vi "IO Manager.vi"(5 "Reentrant?":bool, 7 "Actions":T4, 11 "Mutex Name":string) -> (3 "Success?":bool)   [LabVIEW 2021]
uses:
  <vilib>/myRIO/Common/Instrument Driver Framework/Utilities/typedefs/Resource Manager Action Enum.ctl
  <vilib>/myRIO/Common/Instrument Driver Framework/Utilities/typedefs/Mutex Collection.ctl
  <vilib>/myRIO/Common/Instrument Driver Framework/Utilities/typedefs/Named Mutex.ctl
  <vilib>/myRIO/Common/Instrument Driver Framework/Utilities/typedefs/Reentrant Mutex.ctl
panel:
  out "Mutex Collection":T1
  out "error out":errorcluster
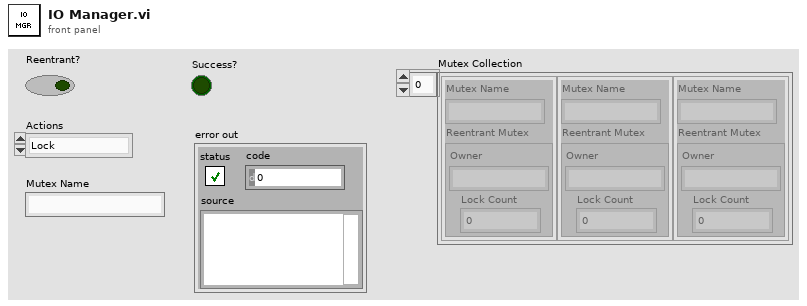
[diagram p1: front panel]
types:
  T1 = typedef "Mutex Collection.ctl" = T2[]
  T2 = typedef "Named Mutex.ctl" = cluster{"Mutex Name":string, "Reentrant Mutex":T3}
  T3 = typedef "Reentrant Mutex.ctl" = cluster{"Owner":string, "Lock Count":u32}
  T4 = typedef "Resource Manager Action Enum.ctl" = enum16{"Lock", "Unlock"}
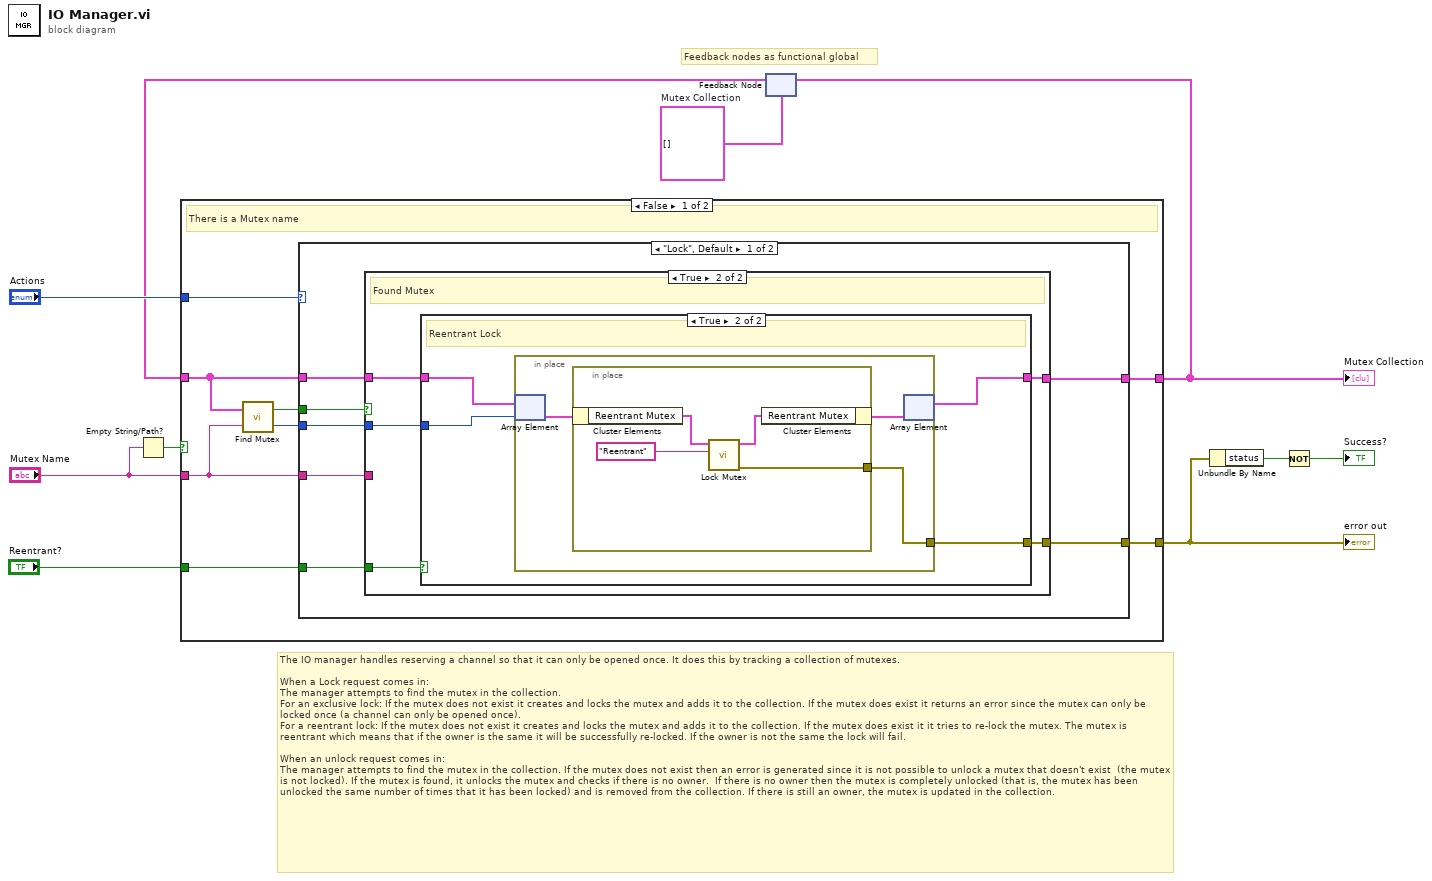
[diagram p0: block diagram]
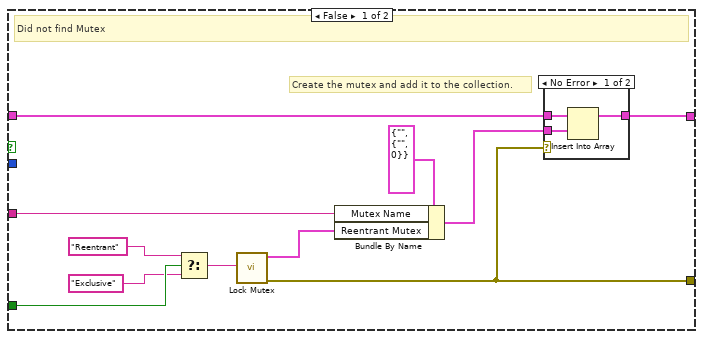
[diagram p2: hidden frame]
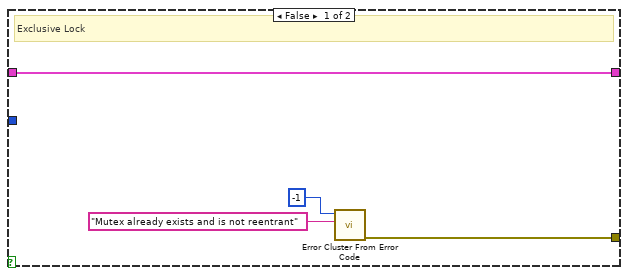
[diagram p4: hidden frame]
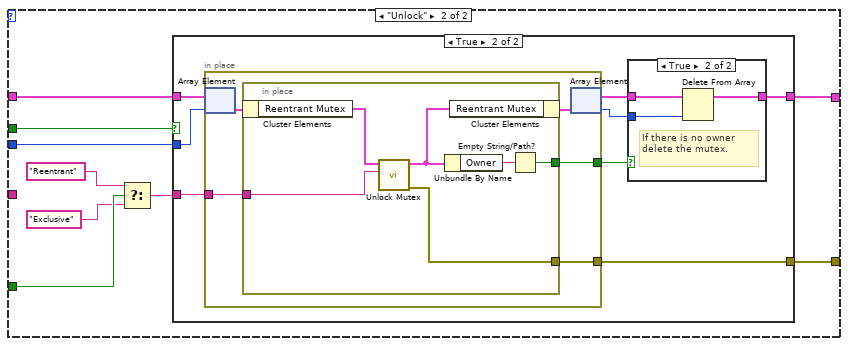
[diagram p5: hidden frame]
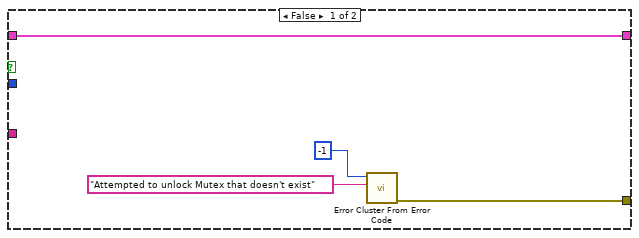
[diagram p6: hidden frame]
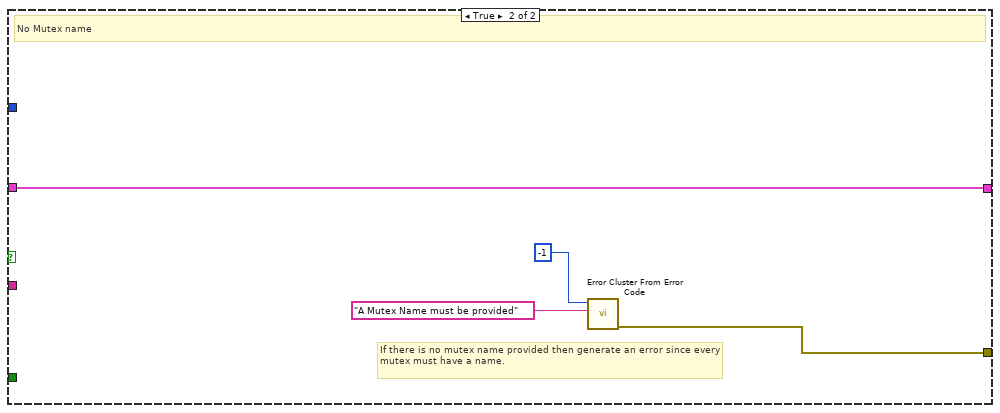
[diagram p8: hidden frame]
diagram:
  w5 = T1 []  # Mutex Collection
  # "The IO manager handles reserving a channel so that it can only be opened once. It does this by tracking a collection of mutexes.\n\nWhen a Lock request comes in:\nThe manager attempts to find the mutex in the collection.\nFor an exclusive lock: If the mutex does not exist it creates and locks the mutex and adds it to the collection. If the mutex does exist it returns an error since the mutex can only be locked once (a channel can only be opened once).\nFor a reentrant lock: If the mutex does not exist it creates and locks the mutex and adds it to the collection. If the mutex does exist it it tries to re-lock the mutex. The mutex is reentrant which means that if the owner is the same it will be successfully re-locked. If the owner is not the same the lock will fail. \n\nWhen an unlock request comes in:\nThe manager attempts to find the mutex in the collection. If the mutex does not exist then an error is generated since it is not possible to unlock a mutex that doesn't exist  (the mutex is not locked). If the mutex is found, it unlocks the mutex and checks if there is no owner.  If there is no owner then the mutex is completely unlocked (that is, the mutex has been unlocked the same number of times that it has been locked) and is removed from the collection. If there is still an owner, the mutex is updated in the collection."
  # "Feedback nodes as functional global"
  n1 = Empty String/Path?(string/path="Mutex Name") -> (empty?=w3:bool)
  n2 = feedback #1(w5) -> (w4:T1)
  n3 = case shown="False" w3 {
    tunnel: "Actions" -> [w18 _]
    tunnel: [w17 w98] -> w9
    tunnel: [w16 w97] -> w6
    tunnel: w4 -> [w14 w97]
    tunnel: "Mutex Name" -> [w11 _]
    tunnel: "Reentrant?" -> [w12 _]
    frame False {
      # "There is a Mutex name"
      n4 = call <vilib>:"Find Mutex.vi"("Mutex Name"=w11, "Mutex Collection"=w14) -> ("Index"=w13:i32, "Found?"=w15:bool)
      n5 = case shown="\"Lock\", Default" w18 {
        tunnel: w14 -> [w25 w68]
        tunnel: [w24 w65] -> w17
        tunnel: [w23 w66] -> w16
        tunnel: w15 -> [w22 w69]
        tunnel: w13 -> [w21 w67]
        tunnel: w12 -> [w20 w64]
        tunnel: w11 -> [w19 _]
        frame "Lock", Default {
          n6 = case shown="True" w22 {
            tunnel: w25 -> [w34 w45]
            tunnel: w21 -> [_ w42]
            tunnel: [w31 w43] -> w24
            tunnel: [w33 w44] -> w23
            tunnel: w19 -> [w30 _]
            tunnel: w20 -> [w29 w41]
            frame False {
              # "Create the mutex and add it to the collection."
              # "Did not find Mutex"
              n7 = Select(t="Reentrant" ("Owner"), s=w29, f="Exclusive" ("Owner")) -> (s? t:f=w26:string)
              n8 = call <vilib>:"Lock Mutex.vi"("Owner"=w26) -> ("error out"=w31:errorcluster, "Mutex Out"=w36:T3)  [unwired: 9 in]
              n9 = Bundle By Name(cluster=T2 {"Mutex Name"="", "Reentrant Mutex"={"Owner"="", "Lock Count"=0}} ("Named Mutex"), "Mutex Name"=w30, "Reentrant Mutex"=w36) -> (w32:T2)
              n10 = case shown="No Error" w31 {
                tunnel: w34 -> [w39 w40]
                tunnel: [w38 w40] -> w33
                tunnel: w32 -> [w37 _]
                frame No Error {
                  n11 = Insert Into Array(array=w39, new element=w37) -> (w38:T1)  [unwired: 1 in]
                }
                frame Error {
                }
              }
            }
            frame True {
              # "Found Mutex"
              n12 = case shown="True" w41 {
                tunnel: w45 -> [w49 w53]
                tunnel: [w49 w52] -> w44
                tunnel: [w46 w51] -> w43
                tunnel: w42 -> [_ w50]
                frame False {
                  # "Exclusive Lock"
                  n13 = call <vilib>:"Error Cluster From Error Code.vi"("error message (\"\")"="Mutex already exists and is not reentrant" ("error message (\"\")"), "error code (0)"=-1) -> ("error out"=w46:errorcluster)  [unwired: 7 in]
                }
                frame True {
                  # "Reentrant Lock"
                  n14 = in-place {
                    in-place-border: [w56] -> w51
                    n15 = in-place-array #2(w53, w50) -> (w55:T2)
                    n16 = in-place {
                      in-place-border: [w60] -> w56
                      n17 = in-place-cluster #3(w55) -> ("Reentrant Mutex"=w59:T3)
                      n18 = call <vilib>:"Lock Mutex.vi"("Owner"="Reentrant", "Mutex In"=w59) -> ("error out"=w60:errorcluster, "Mutex Out"=w58:T3)  [unwired: 8 in]
                      n19 = in-place-cluster #3("Reentrant Mutex"=w58) -> (w54:T2)
                    }
                    n20 = in-place-array #2(w54) -> (w52:T1)  [unwired: 1 out]
                  }
                }
              }
            }
          }
        }
        frame "Unlock" {
          n21 = Select(t="Reentrant", s=w64, f="Exclusive") -> (s? t:f=w61:string)
          n22 = case shown="True" w69 {
            tunnel: w68 -> [w70 w79]
            tunnel: w67 -> [_ w78]
            tunnel: [w70 w80] -> w66
            tunnel: [w73 w75] -> w65
            tunnel: w61 -> [_ w74]
            frame False {
              n23 = call <vilib>:"Error Cluster From Error Code.vi"("error message (\"\")"="Attempted to unlock Mutex that doesn't exist" ("error message (\"\")"), "error code (0)"=-1) -> ("error out"=w73:errorcluster)  [unwired: 7 in]
            }
            frame True {
              n24 = in-place {
                in-place-border: [w86] -> w81
                in-place-border: [w83] -> w75
                in-place-border: w74 -> [w82]
                n25 = in-place-array #4(w79, w78) -> (w85:T2)
                n26 = in-place {
                  in-place-border: [w91] -> w86
                  in-place-border: [w88] -> w83
                  in-place-border: w82 -> [w87]
                  n27 = in-place-cluster #5(w85) -> ("Reentrant Mutex"=w90:T3)
                  n28 = call <vilib>:"Unlock Mutex.vi"("Owner"=w87, "Mutex In"=w90) -> ("error out"=w88:errorcluster, "Mutex Out"=w89:T3)  [unwired: 8 in]
                  n29 = Unbundle By Name(w89) -> ("Owner"=w92:string)
                  n30 = in-place-cluster #5("Reentrant Mutex"=w89) -> (w84:T2)
                  n31 = Empty String/Path?(string/path=w92) -> (empty?=w91:bool)
                }
                n32 = in-place-array #4(w84) -> (w77:T1, w76:i32)
              }
              n33 = case shown="True" w81 {
                tunnel: w77 -> [w93 w96]
                tunnel: w76 -> [_ w95]
                tunnel: [w93 w94] -> w80
                frame False {
                }
                frame True {
                  # "If there is no owner delete the mutex."
                  n34 = Delete From Array(array=w96, index=w95) -> (array with subset deleted=w94:T1)  [unwired: 1 in, 1 out]
                }
              }
            }
          }
        }
      }
    }
    frame True {
      # "If there is no mutex name provided then generate an error since every mutex must have a name."
      # "No Mutex name"
      n35 = call <vilib>:"Error Cluster From Error Code.vi"("error message (\"\")"="A Mutex Name must be provided" ("error message (\"\")"), "error code (0)"=-1) -> ("error out"=w98:errorcluster)  [unwired: 7 in]
    }
  }
  "error out" <- w9
  "Mutex Collection" <- w6
  n36 = feedback-in #1(w6) -> ()
  n37 = Unbundle By Name(w9) -> ("status"=w8:bool)
  n38 = Not(x=w8) -> (.not. x?=→"Success?":bool)
